vi "Main.vi"() -> ()   [LabVIEW 2017]
uses:
  Temp_class/Temp.lvclass
panel:
  out "Temperature Sample Standard Deviation":dbl
  out "Temperature Sample Average":dbl
  in  "Temperature Channel Numbers (Zero Based)":i32[](array[numeric])
  out "Temperature Channel Readings":dbl[](array[numeric])
  out "Temperature Readings":dbl[](array[numeric])
  in  "Quit Program":bool
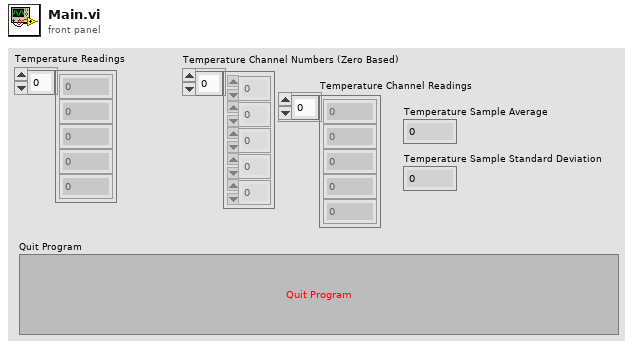
[diagram p1: front panel]
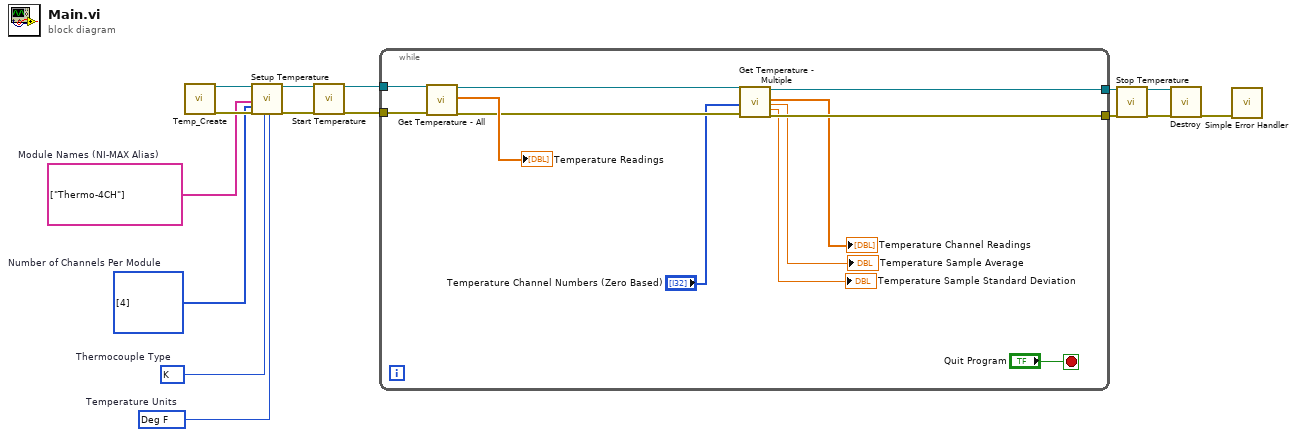
[diagram p0: block diagram]
diagram:
  w10 = u32[] [4]  # Number of Channels Per Module
  w11 = string[] ["Thermo-4CH"]  # Module Names (NI-MAX Alias)
  w12 = 10144 items=["Deg C"=10143, "Deg F"=10144, "Kelvins"=10325, "Deg R"=10145, "From Custom Scale"=10065]  # Temperature Units
  w1 = 10073 items=["J"=10072, "K"=10073, "N"=10077, "R"=10082, "S"=10085, "T"=10086, "B"=10047, "E"=10055]  # Thermocouple Type
  n1 = call "Temp_Create.vi"() -> ("reference out"=w15:refnum<class "Temp.lvclass">, "error out"=w14:errorcluster)  [unwired: 18 in]
  n2 = call-dynamic "Setup Temperature.vi"("reference in"=w15, "Module Names (NI-MAX Alias)"=w11, "Number of Channels Per Module"=w10, "error in (no error)"=w14, "Thermocouple Type"=w1, "Temperature Units"=w12) -> ("reference out"=w9:refnum<class "Temp.lvclass">, "error out"=w8:errorcluster)  [unwired: 12 in]
  n3 = call-dynamic "Start Temperature.vi"("reference in"=w9, "error in (no error)"=w8) -> ("reference out"=w7:refnum<class "Temp.lvclass">, "error out"=w6:errorcluster)  [unwired: 16 in]
  n4 = while {
    tunnel: w7 -> [w26]
    tunnel: w6 -> [w25]
    tunnel: [w22] -> w3
    tunnel: [w20] -> w2
    stop <- "Quit Program" stop-if-true
    n5 = call-dynamic "Get Temperature - All.vi"("reference in"=w26, "error in (no error)"=w25) -> ("reference out"=w23:refnum<class "Temp.lvclass">, "Temperature Readings"=→"Temperature Readings":dbl[], "error out"=w21:errorcluster)  [unwired: 13 in, 2 out]
    n6 = call-dynamic "Get Temperature - Multiple.vi"("reference in"=w23, "Temperature Channel Numbers (Zero Based)"="Temperature Channel Numbers (Zero Based)", "error in (no error)"=w21) -> ("reference out"=w22:refnum<class "Temp.lvclass">, "Temperature Channel Readings"=→"Temperature Channel Readings":dbl[], "Temperature Average Among Channels"=→"Temperature Sample Average":dbl, "Temperature Standard Deviation Among Channels"=→"Temperature Sample Standard Deviation":dbl, "error out"=w20:errorcluster)  [unwired: 12 in]
  }
  n7 = call-dynamic "Stop Temperature.vi"("reference in"=w3, "error in (no error)"=w2) -> ("reference out"=w5:refnum<class "Temp.lvclass">, "error out"=w4:errorcluster)  [unwired: 16 in]
  n8 = call-dynamic "Destroy.vi"("reference in"=w5, "error in (no error)"=w4) -> ("error out"=w13:errorcluster)  [unwired: 16 in, 1 out]
  n9 = call <vilib>:"Simple Error Handler.vi"("error in (no error)"=w13) -> ()  [unwired: 4 in, 5 out]
